vi "Configure Marker Frequency Counter.vi"(8 "error in (no error)":errorcluster, 9 "Active Marker (1: Marker 1)":i32(ring)=1 items=["Marker 1"=1, "Marker 2"=2, "Marker 3"=3, "Marker 4"=4, "Marker 5"=5, "Marker 6"=6], 10 "Enable Frequency Counter (T: Enable)":bool=TRUE, 11 "VISA resource name":refnum<visa-resource-name>) -> (0 "error out":errorcluster, 3 "VISA resource name out":refnum<visa-resource-name>)   [LabVIEW 2022 SP3, in "Agilent N934X Series.lvlib"]
doc: "Configures the marker frequency counter settings on the spectrum analyzer."
uses:
  <instrlib>/Agilent N934X Series/Agilent N934X Series.lvlib
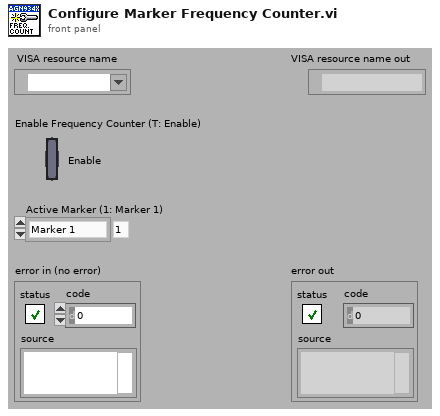
[diagram p1: front panel]
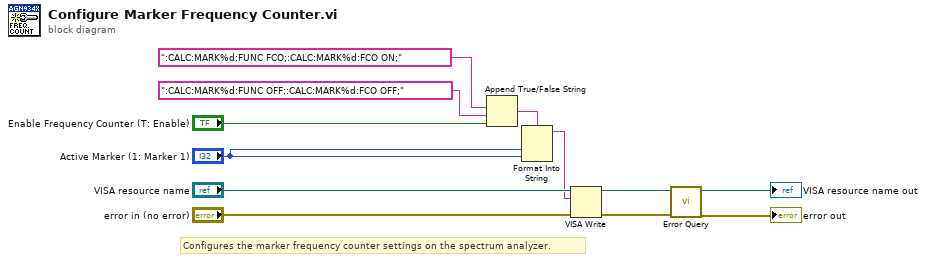
[diagram p0: block diagram]
diagram:
  # "Configures the marker frequency counter settings on the spectrum analyzer."
  n1 = Append True/False String(1:"Enable Frequency Counter (T: Enable)", 2:":CALC:MARK%d:FUNC OFF;:CALC:MARK%d:FCO OFF;", 3:":CALC:MARK%d:FUNC FCO;:CALC:MARK%d:FCO ON;") -> (0:w3:string)  [unwired: 1 in]
  n2 = Format Into String(format string=w3, "Active Marker (1: Marker 1)", "Active Marker (1: Marker 1)") -> (resulting string=w1:string)  [unwired: 2 in, 1 out]
  n3 = VISA Write(VISA resource name="VISA resource name", write buffer=w1, error in (no error)="error in (no error)") -> (VISA resource name out=w10:refnum<visa-resource-name>, error out=w9:errorcluster)  [unwired: 1 out]
  n4 = call <instrlib>:"Error Query.vi"("error in (no error)"=w9, "VISA resource name"=w10) -> ("error out"=→"error out":errorcluster, "VISA resource name out"=→"VISA resource name out":refnum<visa-resource-name>)  [unwired: 6 in, 2 out]
